vi "OnValueChange_AnyKey.vi"(8 "error in (no error)":errorcluster, 11 "PongDemo in":refnum<class "PongDemo.lvclass">) -> (0 "error out":errorcluster, 3 "PongDemo out":refnum<class "PongDemo.lvclass">)   [LabVIEW 2019, in "RT_Game.lvlib" / "PongDemo.lvclass"]
uses:
  PongDemo.lvclass
  Pong/Pong.lvclass
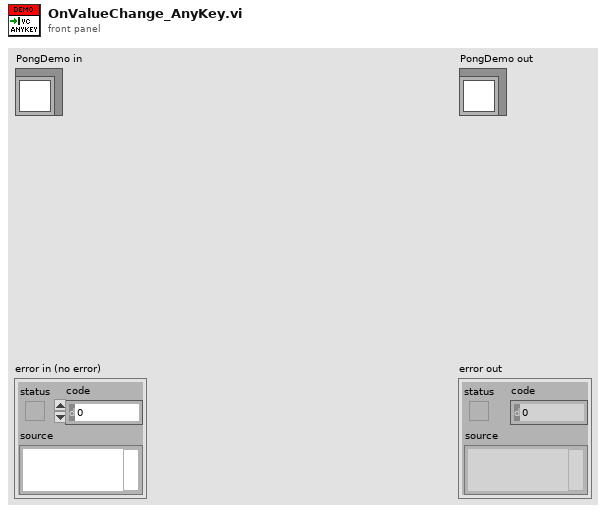
[diagram p1: front panel]
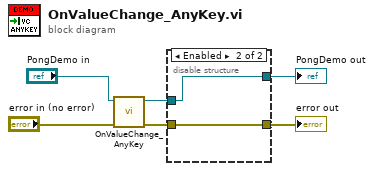
[diagram p0: block diagram]
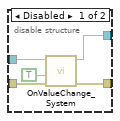
[diagram p2: hidden frame]
diagram:
  n1 = call-parent "OnValueChange_AnyKey.vi"("error in (no error)"="error in (no error)", "Game in"="PongDemo in") -> ("error out"=w6:errorcluster, "Game out"=w2:refnum<class "PongDemo.lvclass">)  [unwired: 8 in]
  n2 = disable-structure shown="Enabled" {
    disable-tunnel: w6 -> [w11 w12]
    disable-tunnel: [w10 w12] -> w3
    disable-tunnel: w2 -> [w9 w13]
    disable-tunnel: [w8 w13] -> w1
    frame Disabled {
      n3 = call-dynamic "OnValueChange_System.vi"("error in (no error)"=w11, "Value"=TRUE, "Game in"=w9) -> ("error out"=w10:errorcluster, "Game out"=w8:refnum<class "PongDemo.lvclass">)  [unwired: 7 in]
    }
    frame Enabled {
    }
  }
  "error out" <- w3
  "PongDemo out" <- w1
